vi "Get Bucket Versioning.vi"(8 "error in (no error)":errorcluster, 11 "Bucket in":refnum<class "Bucket.lvclass">) -> (0 "error out":errorcluster, 1 "MFA Delete":T1, 2 "Status":T2, 3 "Bucket out":refnum<class "Bucket.lvclass">)   [LabVIEW 2015, in "NI_AWS_S3.lvlib" / "Bucket.lvclass"]
uses:
  Bucket.lvclass
  Versioning Status.ctl
  MFA Delete.ctl
  Core/HTTP Request/Region handling.ctl
  Core/HTTP Request/Request Options.ctl
  Core/HTTP Request/Name Value Pair.ctl
  Core/HTTP Request/URL formatting.ctl
  Bucket.lvclass/Bucket.ctl
  Read Name.vi
  Core/HTTP Request/HTTP Request.lvclass
  NI_AWS_S3.lvlib
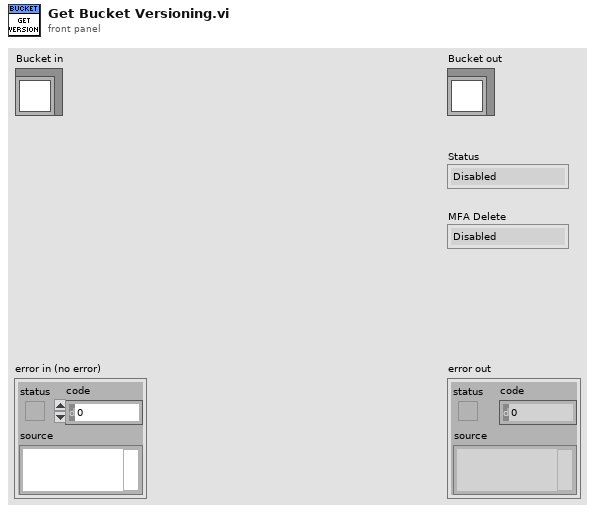
[diagram p1: front panel]
types:
  T1 = typedef "NI_AWS_S3.lvlib/Bucket.lvclass/MFA Delete.ctl" = enum16{"Disabled", "Enabled"}
  T2 = typedef "NI_AWS_S3.lvlib/Bucket.lvclass/Versioning Status.ctl" = enum16{"Disabled", "Suspended", "Enabled"}
  T3 = typedef "NI_AWS_Core.lvlib/HTTP Request.lvclass/Name Value Pair.ctl" = cluster{"name":string, "value":string}
  T4 = typedef "NI_AWS_Core.lvlib/HTTP Request.lvclass/Request Options.ctl" = cluster{"request headers":T3[], "request parameters":T3[], "request body":string, "region handling":T5, "URL formatting":T6}
  T5 = typedef "NI_AWS_S3.lvlib/Region handling.ctl" = enum16{"use region everywhere", "use region (authentication only)", "use region (URL only)", "ignore region everwhere"}
  T6 = typedef "NI_AWS_S3.lvlib/URL formatting.ctl" = enum16{"region-", "region."}
  T7 = typedef "NI_AWS_Core.lvlib/HTTP Request.lvclass/Response.ctl" = cluster{"Headers":string, "Body":string}
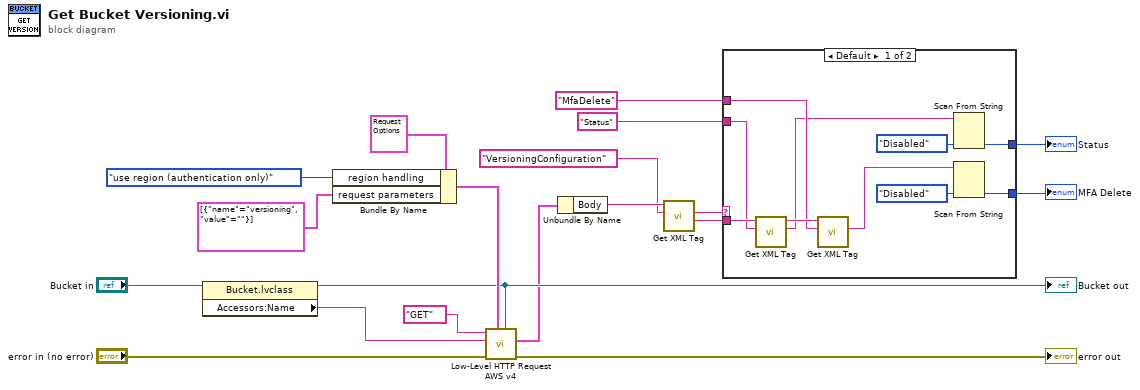
[diagram p0: block diagram]
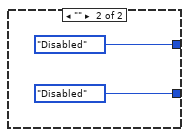
[diagram p2: hidden frame]
diagram:
  n1 = property class="Bucket.lvclass"(reference="Bucket in") -> (reference out=w13:refnum<class "Bucket.lvclass">, "Accessors:Name"=w18:string)  [unwired: 1 in, 1 out]
  "Bucket out" <- w13
  n2 = Bundle By Name(cluster=T4 {"request headers"=[], "request parameters"=[], "request body"="", "region handling"=enum."use region everywhere", "URL formatting"=enum."region."} ("Request Options"), "region handling"=Region_handling."use region (authentication only)", "request parameters"=T3[] [{"name"="versioning", "value"=""}]) -> (w15:T4)
  n3 = call "Low-Level HTTP Request AWS v4.vi"("AWS Core"=w13, "Request Options"=w15, "error in (no error)"="error in (no error)", "URL Prefix"=w18, "HTTP-Verb"="GET") -> ("error out"=→"error out":errorcluster, "Response"=w8:T7)  [unwired: 4 in, 1 out]
  n4 = Unbundle By Name(w8) -> ("Body"=w9:string)
  n5 = call "Get XML Tag.vi"("Tag name"="VersioningConfiguration", "XML String in"=w9) -> ("Remaining string"=w5:string, "Tag value"=w6:string)  [unwired: 5 in, 3 out]
  n6 = case shown="Default" w6 {
    tunnel: w5 -> [w29 _]
    tunnel: [w21 Versioning_Status."Disabled" ("Status")] -> w4
    tunnel: [w22 MFA_Delete."Disabled" ("MFA Delete")] -> w3
    tunnel: "Status" ("Tag name") -> [w28 _]
    tunnel: "MfaDelete" ("Tag name") -> [w26 _]
    frame Default {
      n7 = call "Get XML Tag.vi"("Tag name"=w28, "XML String in"=w29) -> ("Tag value"=w25:string, "XML String dup"=w27:string)  [unwired: 5 in, 3 out]
      n8 = call "Get XML Tag.vi"("Tag name"=w26, "XML String in"=w27) -> ("Tag value"=w20:string)  [unwired: 5 in, 4 out]
      n9 = Scan From String(input string=w25, default 1=Versioning_Status."Disabled" ("Status")) -> (output 1=w21:T2)  [unwired: 3 in, 3 out]
      n10 = Scan From String(input string=w20, default 1=MFA_Delete."Disabled" ("MFA Delete")) -> (output 1=w22:T1)  [unwired: 3 in, 3 out]
    }
    frame "" {
    }
  }
  "Status" <- w4
  "MFA Delete" <- w3
